vi "Do.vi"(8 "error in (no error)":errorcluster, 9 "File Path":path, 10 "File Writer in":refnum<class "File Writer.lvclass">, 11 "File Post Action in":refnum<class "File Post Action.lvclass">) -> (0 "error out":errorcluster, 2 "File Writer out":refnum<class "File Writer.lvclass">)   [LabVIEW 2020, in "File Writer.lvlib" / "File Post Action.lvclass"]
doc: "Perform a Post file Action."
uses:
  File Post Action.lvclass
  File Writer.lvclass
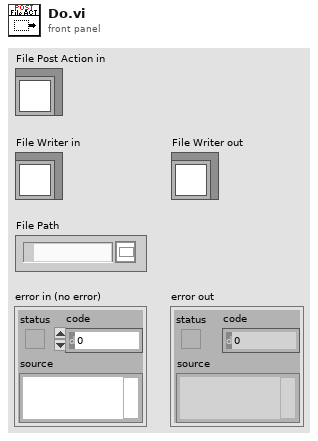
[diagram p1: front panel]
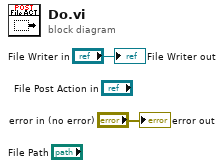
[diagram p0: block diagram]
diagram:
  "error out" <- "error in (no error)"
  "File Writer out" <- "File Writer in"
